vi "Exemple_Preprocessing_minmax_scale.vi"() -> ()   [LabVIEW 2020]
panel:
  out "Data":T1
  out "error out":errorcluster
  in  "X":string[][](array[string])=[["-1", "2"], ["-0,5", "6"], ["0", "10"], ["1", "18"]]
  in  "error in":errorcluster caption="entrée d'erreur"
  in  "minmax_scale":T2={"feature_range"={"min"=0.0, "max"=1.0}, "axis"=0, "copy"=TRUE}
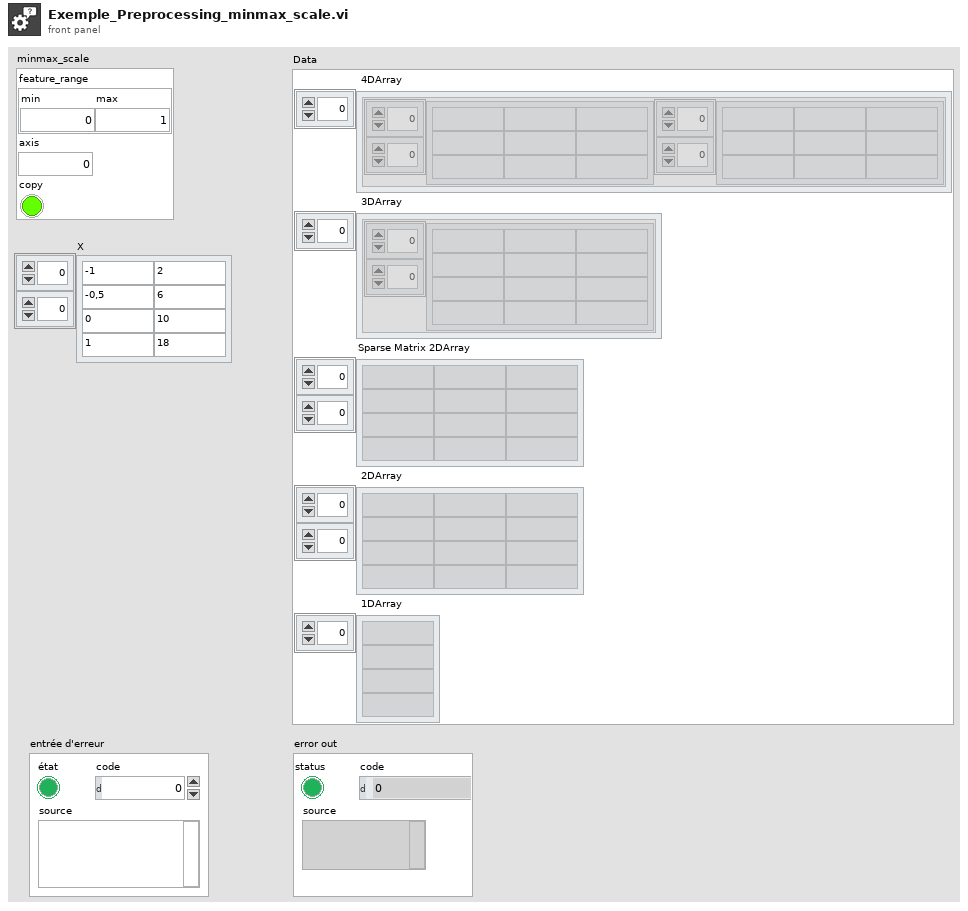
[diagram p1: front panel]
types:
  T1 = cluster{" 4DArray":cluster{"1":string[][], "2":string[][]}[], " 3DArray":cluster{"Tableau":string[][]}[], "Sparse Matrix 2DArray":string[][], " 2DArray":string[][], " 1DArray":string[]}
  T2 = cluster{"feature_range":cluster{"min":dbl, "max":dbl}, "axis":i32, "copy":bool}
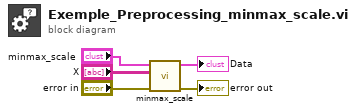
[diagram p0: block diagram]
diagram:
  n1 = call "minmax_scale.vi"("error in"="error in", "X"="X", "minmax_scale"="minmax_scale") -> ("error out"=→"error out":errorcluster, "Data"=→"Data":T1)  [unwired: 7 in]
